vi "read_buff.vi"(0 "buffer":string, 9 "HTTP client handle":T1, 11 "HTTP client error":errorcluster, 12 "array of ranges":cluster{"low":dbl, "high":dbl}[](array[cluster])) -> (4 "client handle out":T1, 6 "queue out":refnum<queue>, 10 "http client error out":errorcluster, 15 "error queue out":errorcluster)   [LabVIEW 2016]
uses:
  <vilib>/httpClient/ClientHandle.ctl
  <vilib>/httpClient/LabVIEWHTTPClient.lvlib
panel:
  out "JSON string":string
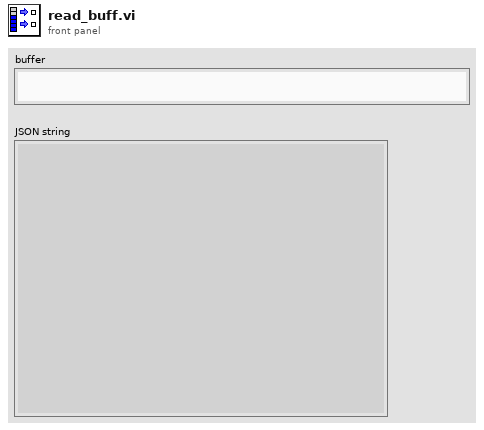
[diagram p1: front panel]
types:
  T1 = typedef "LabVIEWHTTPClient.lvlib/ClientHandle.ctl" = refnum<k1>
  T2 = cluster{"temperature_1":dbl, "temperature_2":dbl, "temperature_3":dbl, "temperature_4":dbl, "pressure":dbl, "current":dbl, "voltage":dbl, "pressure_vacuum":dbl, "rec_volt_out":dbl}
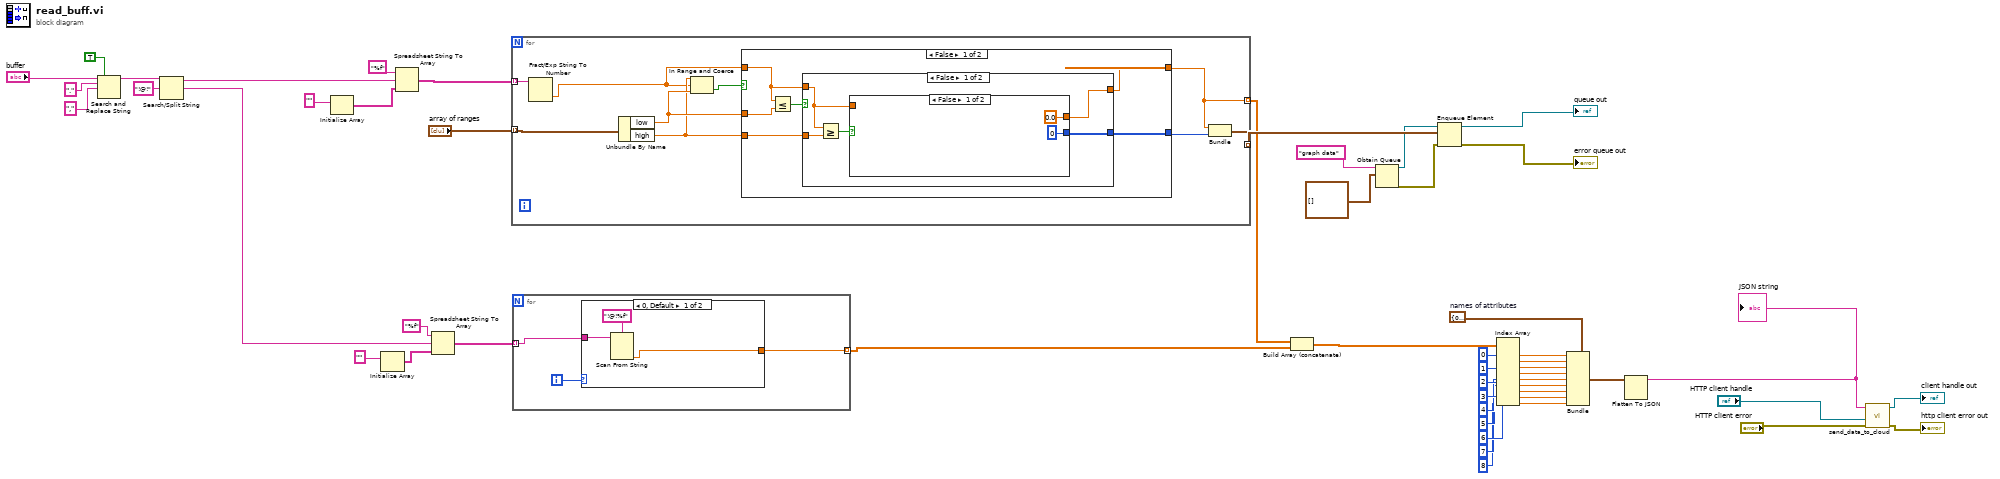
[diagram p0: block diagram]
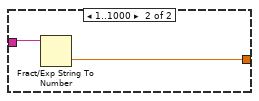
[diagram p2: hidden frame]
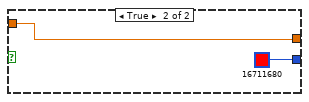
[diagram p3: hidden frame]
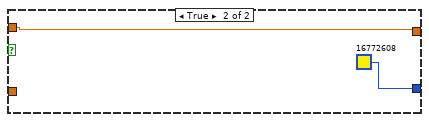
[diagram p4: hidden frame]
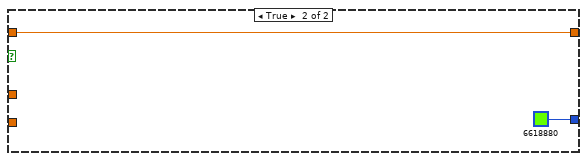
[diagram p5: hidden frame]
diagram:
  w27 = T2 {"temperature_1"=0.0, "temperature_2"=0.0, "temperature_3"=0.0, "temperature_4"=0.0, "pressure"=0.0, "current"=0.0, "voltage"=0.0, "pressure_vacuum"=0.0, "rec_volt_out"=0.0}  # names of attributes
  n1 = Search and Replace String(replace all?=TRUE ("replace all? (F)"), input string="buffer", search string="." ("replace string (\"\")"), replace string="," ("replace string (\"\")")) -> (result string=w25:string)  [unwired: 4 in, 3 out]
  n2 = Search/Split String(string=w25, search string/char (-)="!@!") -> (substring before match=w1:string, match + rest of string=w23:string)  [unwired: 1 in, 1 out]
  n3 = Initialize Array("") -> (w47:string[])  [unwired: 1 in]
  n4 = Initialize Array("") -> (w20:string[])  [unwired: 1 in]
  n5 = Spreadsheet String To Array(format string="%f", spreadsheet string=w1, array type (2D Dbl)=w47) -> (array=w29:string[])  [unwired: 1 in]
  n6 = Spreadsheet String To Array(format string="%f", spreadsheet string=w23, array type (2D Dbl)=w20) -> (array=w19:string[])  [unwired: 1 in]
  n7 = for {
    tunnel: [w56] -> w43 mode=indexing
    tunnel: [w55] -> w13 mode=indexing
    tunnel: w29 -> [w61] mode=indexing
    tunnel: "array of ranges" -> [w54] mode=indexing
    n8 = Fract/Exp String To Number(string=w61) -> (number=w53:dbl)  [unwired: 3 in, 1 out]
    n9 = Unbundle By Name(w54) -> ("low"=w59:dbl, "high"=w57:dbl)
    n10 = In Range and Coerce(upper limit=w57, x=w53, lower limit=w59) -> (In Range?=w60:bool)  [unwired: 1 out]
    n11 = case shown="False" w60 {
      tunnel: w53 -> [w64 w80]
      tunnel: [w63 w80] -> w55
      tunnel: w59 -> [w67 _]
      tunnel: [w65 u32 6618880 ("Round Color Box")] -> w58
      tunnel: w57 -> [w62 _]
      frame False {
        n12 = Less Or Equal?(x=w64, y=w67) -> (x <= y?=w66:bool)
        n13 = case shown="False" w66 {
          tunnel: [w70 u32 16772608 ("Round Color Box")] -> w65
          tunnel: [w68 w77] -> w63
          tunnel: w64 -> [w69 w77]
          tunnel: w62 -> [w71 _]
          frame False {
            n14 = Greater Or Equal?(x=w69, y=w71) -> (x >= y?=w72:bool)
            n15 = case shown="False" w72 {
              tunnel: [u32 0 ("Round Color Box") u32 16711680 ("Round Color Box")] -> w70
              tunnel: [0.0 w75] -> w68
              tunnel: w69 -> [_ w75]
              frame False {
              }
              frame True {
              }
            }
          }
          frame True {
          }
        }
      }
      frame True {
      }
    }
    n16 = Bundle(w55, "Round Color Box"=w58) -> (w56:cluster{dbl, "Round Color Box":u32})  [unwired: 1 in]
  }
  n17 = for {
    tunnel: w19 -> [w83] mode=indexing
    tunnel: [w81] -> w12 mode=indexing
    i -> [w82]
    n18 = case shown="0, Default" w82 {
      tunnel: w83 -> [w86 w88]
      tunnel: [w84 w87] -> w81
      frame 0, Default {
        n19 = Scan From String(format string="!@!%f", input string=w86) -> (output 1=w84:dbl)  [unwired: 3 in, 3 out]
      }
      frame 1..1000 {
        n20 = Fract/Exp String To Number(string=w88) -> (number=w87:dbl)  [unwired: 3 in, 1 out]
      }
    }
  }
  n21 = Build Array (concatenate)(w13, w12) -> (w11:dbl[])
  n22 = Obtain Queue(name (unnamed)="graph data", element data type=cluster{dbl, "Round Color Box":u32}[] []) -> (queue out=w42:refnum<queue>, error out=w32:errorcluster)  [unwired: 3 in, 1 out]
  n23 = Enqueue Element(queue=w42, element=w43, error in (no error)=w32) -> (queue out=→"queue out":refnum<queue>, error out=→"error queue out":errorcluster)  [unwired: 1 in, 1 out]
  n24 = Index Array(array=w11, index #1=0 ("index"), index #2=1 ("index"), index #3=2 ("index"), index #4=3 ("index"), index #5=4 ("index"), index #6=5 ("index"), index #7=6 ("index"), index #8=7 ("index"), index #9=8 ("index")) -> (element #1=w41:dbl, element #2=w40:dbl, element #3=w39:dbl, element #4=w38:dbl, element #5=w37:dbl, element #6=w36:dbl, element #7=w35:dbl, element #8=w34:dbl, element #9=w26:dbl)
  n25 = Bundle(cluster=w27, "temperature_1"=w41, "temperature_2"=w40, "temperature_3"=w39, "temperature_4"=w38, "pressure"=w37, "current"=w36, "voltage"=w35, "pressure_vacuum"=w34, "rec_volt_out"=w26) -> (w33:T2)
  n26 = Flatten To JSON(anything=w33) -> (JSON string=w18:string)  [unwired: 2 in, 1 out]
  "JSON string" <- w18
  n27 = call "send_data_to_cloud.vi"("HTTP client error"="HTTP client error", "HTTP client handle"="HTTP client handle", "buffer"=w18) -> ("http client error out"=→"http client error out":errorcluster, "client handle out"=→"client handle out":T1)  [unwired: 7 in]
